vi "Translate Data.vi"(8 "error in":errorcluster, 10 "BufferIn":string, 11 "V in":refnum<class "V.lvclass">) -> (0 "error out":errorcluster, 2 "DataOut":refnum<class "Data.lvclass">, 3 "V out":refnum<class "V.lvclass">)   [LabVIEW 2013, in "Alicat.lvlib" / "V.lvclass"]
doc: "VI used to translate the data buffer to something meaningful (implementation dependent). This VI must be overridden."
uses:
  V.lvclass
  Reusable/Data/Data.lvclass
  Data/VC/AlicatVCData.lvclass
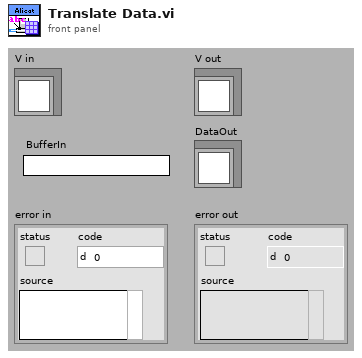
[diagram p1: front panel]
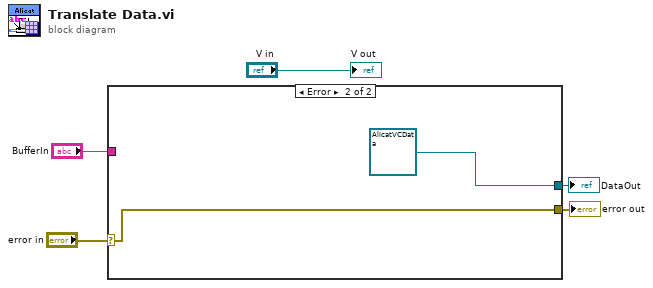
[diagram p0: block diagram]
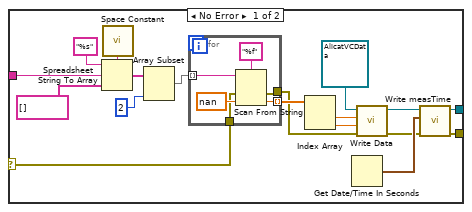
[diagram p2: hidden frame]
diagram:
  n1 = case shown="Error" "error in" {
    selector: "error in" -> [w6 w31]
    tunnel: [w12 w31] -> w5
    tunnel: [w11 refnum<class "AlicatVCData.lvclass"> refnum ("Data out")] -> w4
    tunnel: "BufferIn" -> [w10 _]
    frame No Error {
      n2 = call <vilib>:"Space Constant.vi"() -> ("String"=w22:string)
      n3 = Spreadsheet String To Array(delimiter (Tab)=w22, format string="%s", spreadsheet string=w10, array type (2D Dbl)=string[] []) -> (array=w9:string[])
      n4 = Array Subset(array=w9, length=2) -> (w8:string[])  [unwired: 1 in]
      n5 = for {
        tunnel: w8 -> [w29] mode=indexing
        tunnel: [w26] -> w20 mode=indexing
        tunnel: w6 -> [w25]
        tunnel: [w24] -> w13
        n6 = Scan From String(format string="%f", input string=w29, error in=w25, default 1=sgl nan ("default value 1")) -> (error out=w24:errorcluster, output 1=w26:sgl)  [unwired: 1 in, 2 out]
      }
      n7 = Index Array(array=w20) -> (element #1=w19:sgl, element #2=w18:sgl)  [unwired: 2 in]
      n8 = Get Date/Time In Seconds() -> (seconds since 1Jan1904=w16:timestamp)
      n9 = call "Write Data.vi"("error in (no error)"=w13, "Qsp"=w18, "Q"=w19, "AlicatVData in"=refnum<class "AlicatVCData.lvclass"> refnum) -> ("error out"=w15:errorcluster, "AlicatVData out"=w17:refnum<class "AlicatVCData.lvclass">)  [unwired: 6 in]
      n10 = call "Write measTime.vi"("error in (no error)"=w15, "measTime"=w16, "Data in"=w17) -> ("error out"=w12:errorcluster, "Data out"=w11:refnum<class "AlicatVCData.lvclass">)  [unwired: 7 in]
    }
    frame Error {
    }
  }
  "error out" <- w5
  "DataOut" <- w4
  "V out" <- "V in"
